vi "SecurityCamera.vi"() -> ()   [LabVIEW 2013]
uses:
  <vilib>/vision/Avi.llb/IMAQ AVI2 Refnum.ctl
  <vilib>/vision/Image Controls.llb/IMAQ Image.ctl
  SecurityCameraStates.ctl
  MouseCarousel-Main/GlobalVariables.vi
panel:
  out "Lost Image Count":u32
  out "Acquired Image":T1
  out "Timestamped Image":T1
  out "Shutdown":bool=TRUE
  out "Exit and Close":bool=TRUE
  in  "stop":bool
  in  "Select Mouse ROI":bool
  in  "Show Mouse ROI":bool
  out "Saving Video":bool=TRUE
  out "FPS":dbl
  out "Close Avi File":bool=TRUE
  out "Open Avi File":bool=TRUE
  out "Lost Frames":u32
  out "Last Image Number":u32
  in  "File Path for Mouse Mask":path=path "C:/PassiveRotationTask/MousePositionMask.bmp"
  out "Mouse mask":T1
  out "Mouse Image":T1(plugin-control)
  out "AVI Refnum - Body":T2
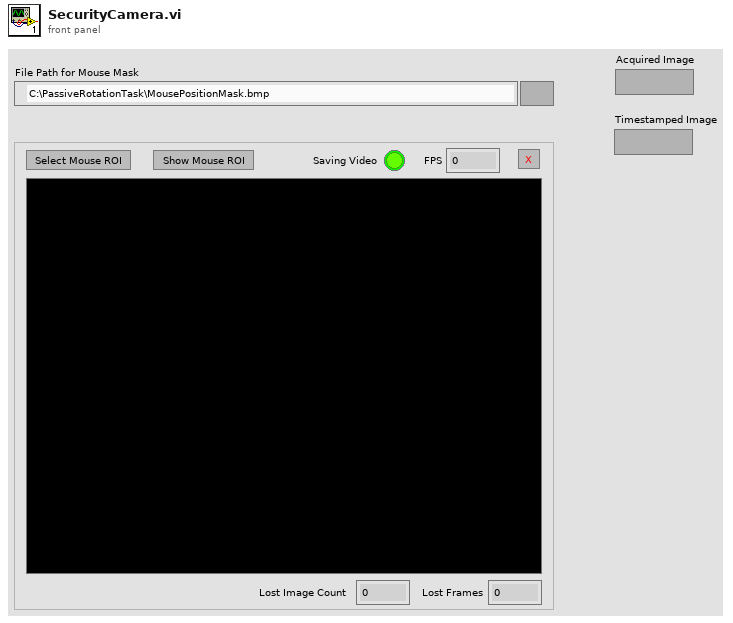
[diagram p1: front panel]
types:
  T1 = typedef "IMAQ Image.ctl" = refnum<image>
  T2 = typedef "IMAQ AVI2 Refnum.ctl" = refnum<k20>
  T3 = typedef "SecurityCameraStates.ctl" = enum16{"Init Security Camera", "Idle", "Process Image", "Acquire Image", "Disconnect Camera", "Exit"}
  T4 = typedef "Image Type" = u32
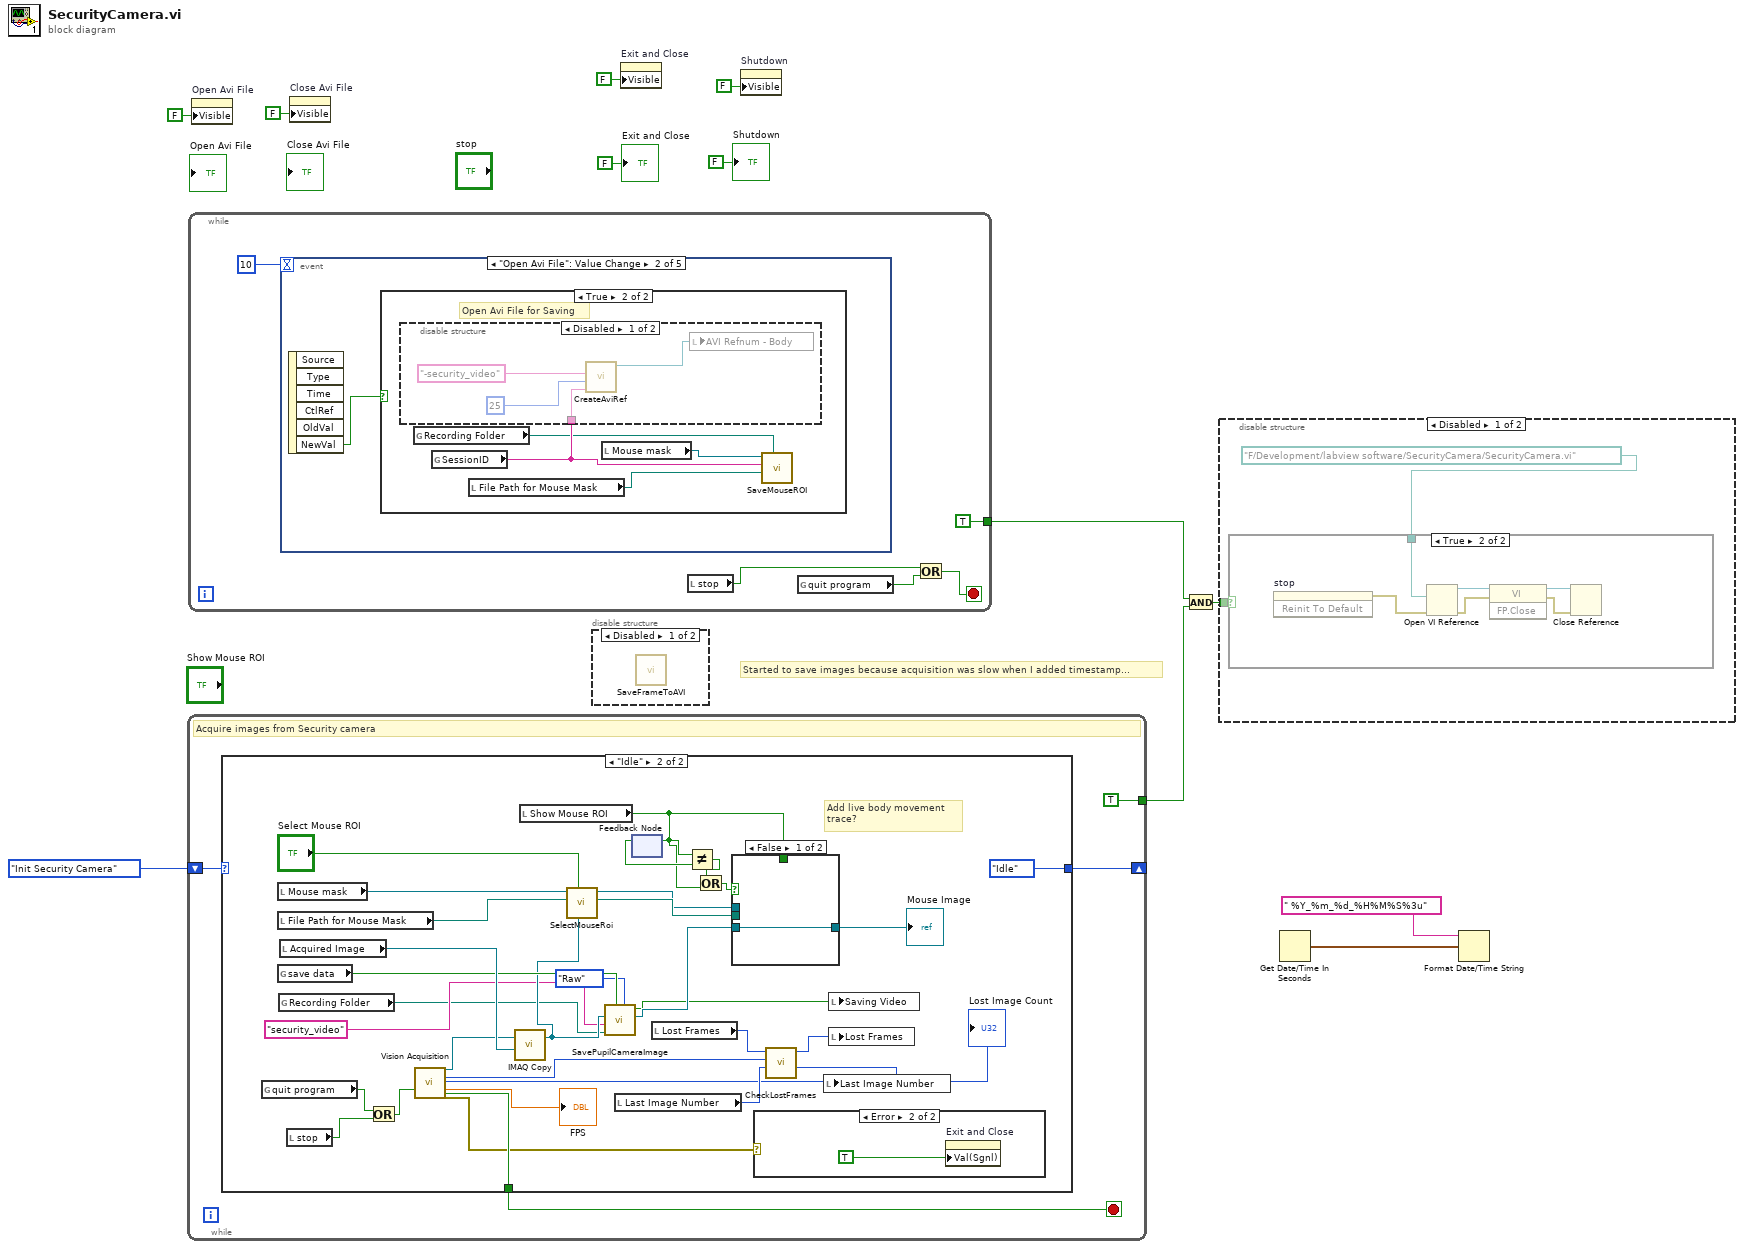
[diagram p0: block diagram]
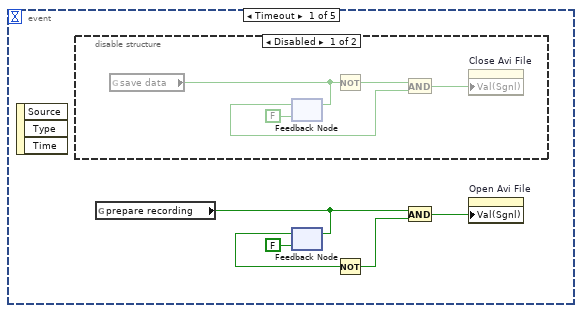
[diagram p5: hidden frame]
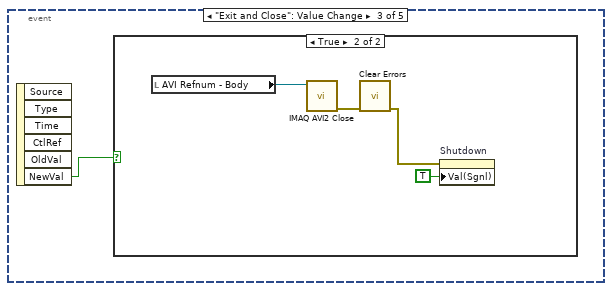
[diagram p9: hidden frame]
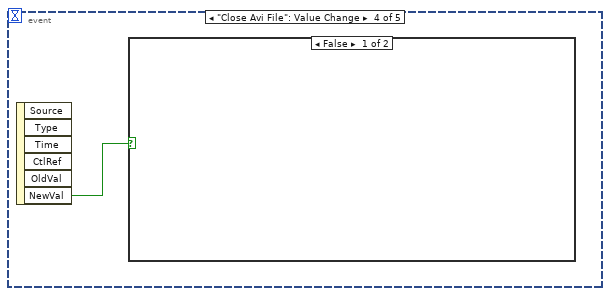
[diagram p11: hidden frame]
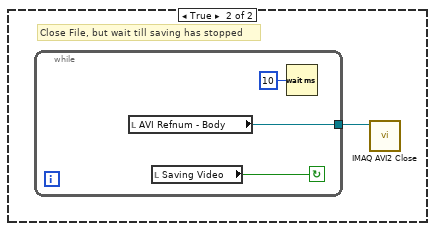
[diagram p12: hidden frame]
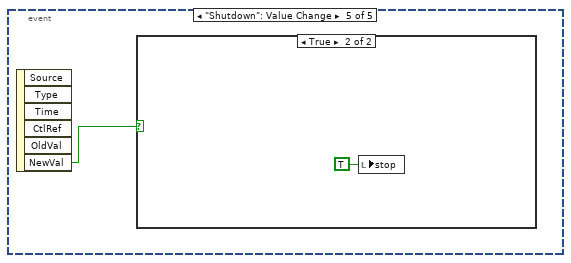
[diagram p13: hidden frame]
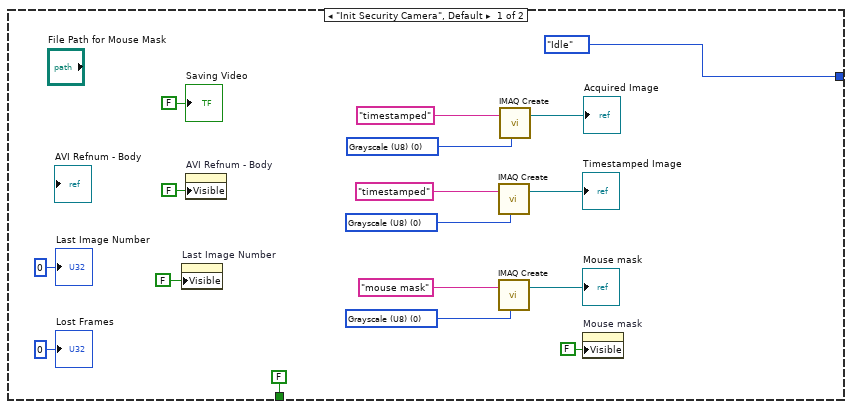
[diagram p15: hidden frame]
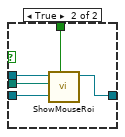
[diagram p16: hidden frame]
diagram:
  # "Started to save images because acquisition was slow when I added timestamp..."
  n1 = while {
    shift-right: [w15] -> _
    shift-left: SecurityCameraStates."Init Security Camera" ("States") -> [w14]
    tunnel: [TRUE] -> w8
    stop <- w16 stop-if-true
    # "Acquire images from Security camera"
    n2 = case shown="\"Idle\"" w14 {
      tunnel: [FALSE ("Stopped") w63] -> w16
      tunnel: [SecurityCameraStates."Idle" ("States") SecurityCameraStates."Idle" ("States")] -> w15
      frame "Init Security Camera", Default {
        w18 = T4 0 items=["Grayscale (U8)", "Grayscale (I16)", "Grayscale (SGL)", "Complex (CSG)", "RGB (U32)", "HSL (U32)", "RGB (U64)", "Grayscale (U16)"] ("Image Type")
        w21 = T4 0 items=["Grayscale (U8)", "Grayscale (I16)", "Grayscale (SGL)", "Complex (CSG)", "RGB (U32)", "HSL (U32)", "RGB (U64)", "Grayscale (U16)"] ("Image Type")
        w25 = T4 0 items=["Grayscale (U8)", "Grayscale (I16)", "Grayscale (SGL)", "Complex (CSG)", "RGB (U32)", "HSL (U32)", "RGB (U64)", "Grayscale (U16)"] ("Image Type")
        n3 = property on="Last Image Number" class="DigNum (strict)"("Visible"=FALSE) -> ()  [unwired: 2 in, 2 out]
        n4 = property on="AVI Refnum - Body" class="IMAQAVI (strict)"("Visible"=FALSE) -> ()  [unwired: 2 in, 2 out]
        n5 = call "IMAQ Create"("Image Name"="timestamped", "Image Type"=w21) -> ("New Image"=→"Timestamped Image":T1)  [unwired: 3 in, 1 out]
        n6 = call "IMAQ Create"("Image Name"="mouse mask", "Image Type"=w25) -> ("New Image"=→"Mouse mask":T1)  [unwired: 3 in, 1 out]
        n7 = call "IMAQ Create"("Image Name"="timestamped", "Image Type"=w18) -> ("New Image"=→"Acquired Image":T1)  [unwired: 3 in, 1 out]
        n8 = property on="Mouse mask" class="IMAQImage (strict)"("Visible"=FALSE) -> ()  [unwired: 2 in, 2 out]
        "Last Image Number" <- u32 0 ("Last Image number 2")
        "Lost Frames" <- u32 0 ("LostFrames 2")
        "Saving Video" <- FALSE ("Saving Security Video")
      }
      frame "Idle" {
        # "Add live body movement\ntrace?"
        n9 = global read "GlobalVariables.vi" "quit program"() -> (w52:bool)
        n10 = local read "Mouse mask"() -> (w59:T1)
        n11 = local read "File Path for Mouse Mask"() -> (w61:path)
        n12 = global read "GlobalVariables.vi" "save data"() -> (w41:bool)
        n13 = global read "GlobalVariables.vi" "Recording Folder"() -> (w37:path)
        n14 = local read "Acquired Image"() -> (w46:T1)
        n15 = local read "stop"() -> (w51:bool)
        n16 = Or(x=w52, y=w51) -> (x .or. y?=w50:bool)
        n17 = call "Vision Acquisition"("Stop (F)"=w50) -> ("Image Out"=w42:T1, "Image Number"=w55:i32, "Lost Image Count"=→"Lost Image Count":u32, "Frame Rate"=→"FPS":dbl, "Stopped"=w63:bool, "error out"=w49:errorcluster)  [unwired: 20 in, 1 out]
        n18 = call "IMAQ Copy"("Image Dst"=w46, "Image Src"=w42) -> ("Image Dst Out"=w39:T1)  [unwired: 4 in, 1 out]
        n19 = local read "Show Mouse ROI"() -> (w43:bool)
        n20 = call "SelectMouseRoi.vi"("Refnum in"=w39, "Select mouse"="Select Mouse ROI", "File Path for Mouse Mask"=w61, "MouseRoi"=w59) -> ()  [unwired: 7 in, 1 out]
        n21 = call "SavePupilCameraImage.vi"("Save Format"=enum16{"Png", "Raw"}."Raw", "Save Image?"=w41, "Block Folder"=w37, "Subfolder"="security_video", "Refnum in"=w39) -> ("Refnum out (duplicate)"=w40:T1, "ImageSaved"=w36:bool)  [unwired: 5 in]
        n22 = local read "Last Image Number"() -> (w54:u32)
        n23 = feedback-in #1(w43) -> ()
        n24 = feedback #1() -> (w47:bool)  [unwired: 1 in]
        n25 = local read "Lost Frames"() -> (w56:u32)
        n26 = Not Equal?(x=w43, y=w47) -> (x != y?=w45:bool)
        n27 = Or(x=w45, y=w43) -> (x .or. y?=w44:bool)
        n28 = case shown="False" w44 {
          tunnel: w61 -> [_ w69]
          tunnel: w40 -> [w64 w68]
          tunnel: w59 -> [_ w67]
          tunnel: [w64 w66] -> w48
          tunnel: w43 -> [_ w65]
          frame False {
          }
          frame True {
            n29 = call "ShowMouseRoi.vi"("Refnum Image In"=w68, "Show mouse selection"=w65, "File Path for Mouse Mask"=w69, "Refnum MouseROI"=w67) -> ("Refnum Image out"=w66:T1)  [unwired: 7 in]
          }
        }
        "Mouse Image" <- w48
        n30 = case shown="Error" w49 {
          frame No Error {
          }
          frame Error {
            n31 = property on="Exit and Close" class="Bool (strict)"("Val(Sgnl)"=TRUE ("Value (Signaling)")) -> ()  [unwired: 2 in, 2 out]
          }
        }
        n32 = call "CheckLostFrames.vi"("Last Image number"=w54, "Image Number"=w55, "LostFrames in"=w56) -> ("Last Image Number"=w57:u32, "LostFrames out"=w58:u32)  [unwired: 5 in, 2 out]
        n33 = local write "Last Image Number"(w57) -> ()
        n34 = local write "Saving Video"(w36) -> ()
        n35 = local write "Lost Frames"(w58) -> ()
      }
    }
  }
  n36 = while {
    tunnel: [TRUE] -> w9
    stop <- w72 stop-if-true
    n37 = event shown="[1] \"Open Avi File\": Value Change" {
      selector: _ -> [_ _ _ _ _]
      dyn-events: _ -> [_ _ _ _ _]
      timeout: 10 -> [_ _ _ _ _]
      event Timeout {
        n38 = event-data() -> ()  [unwired: 1 in, 3 out]
        n39 = disable-structure shown="Disabled" {
          frame Disabled {
            n40 = global read "GlobalVariables.vi" "save data"() -> (w84:bool)
            n41 = feedback #2(FALSE ("save data")) -> (w82:bool)
            n42 = feedback-in #2(w84) -> ()
            n43 = Not(x=w84) -> (.not. x?=w83:bool)
            n44 = And(x=w83, y=w82) -> (x .and. y?=w81:bool)
            n45 = property on="Close Avi File" class="Bool (strict)"("Val(Sgnl)"=w81) -> ()  [unwired: 2 in, 2 out]
          }
          frame Enabled {
          }
        }
        n46 = global read "GlobalVariables.vi" "prepare recording"() -> (w78:bool)
        n47 = feedback #3(FALSE ("save data")) -> (w77:bool)
        n48 = feedback-in #3(w78) -> ()
        n49 = Not(x=w77) -> (.not. x?=w76:bool)
        n50 = And(x=w78, y=w76) -> (x .and. y?=w79:bool)
        n51 = property on="Open Avi File" class="Bool (strict)"("Val(Sgnl)"=w79) -> ()  [unwired: 2 in, 2 out]
      }
      event "Open Avi File": Value Change {
        n52 = event-data() -> ("NewVal"=w86:bool)  [unwired: 1 in, 5 out]
        n53 = case shown="True" w86 {
          frame False {
          }
          frame True {
            # "Open Avi File for Saving"
            n54 = global read "GlobalVariables.vi" "Recording Folder"() -> (w87:path)
            n55 = global read "GlobalVariables.vi" "SessionID"() -> (w88:string)
            n56 = disable-structure shown="Disabled" {
              disable-tunnel: w88 -> [w91 _]
              frame Disabled {
                n57 = call "CreateAviRef.vi"("sessionID"=w91, "Framerate"=u32 25, "Filename prefix"="-security_video") -> ("Refnum out"=w93:T2, "Block folder"=w92:path)  [unwired: 7 in]
                n58 = local write "AVI Refnum - Body"(w93) -> ()
              }
              frame Enabled {
              }
            }
            n59 = local read "File Path for Mouse Mask"() -> (w90:path)
            n60 = local read "Mouse mask"() -> (w89:T1)
            n61 = call "SaveMouseROI.vi"("BlockFolderPath"=w87, "File Path for Mouse Mask"=w90, "sessionID"=w88, "MouseRoi Refnum in"=w89) -> ()  [unwired: 8 in]
          }
        }
      }
      event "Exit and Close": Value Change {
        n62 = event-data() -> ("NewVal"=w96:bool)  [unwired: 1 in, 5 out]
        n63 = case shown="True" w96 {
          frame False {
          }
          frame True {
            n64 = local read "AVI Refnum - Body"() -> (w100:T2)
            n65 = call "IMAQ AVI2 Close"("AVI Refnum"=w100) -> ("error out"=w99:errorcluster)  [unwired: 10 in]
            n66 = call <vilib>:"Clear Errors.vi"("error in (no error)"=w99) -> ("error out"=w98:errorcluster)  [unwired: 6 in]
            n67 = property on="Shutdown" class="Bool (strict)"(error in=w98, "Val(Sgnl)"=TRUE ("Value (Signaling)")) -> ()  [unwired: 1 in, 2 out]
          }
        }
      }
      event "Close Avi File": Value Change {
        n68 = event-data() -> ("NewVal"=w101:bool)  [unwired: 1 in, 5 out]
        n69 = case shown="False" w101 {
          frame False {
          }
          frame True {
            # "Close File, but wait till saving has stopped"
            n70 = while {
              tunnel: [w103] -> w102
              stop <- w105 continue-if-true
              n71 = local read "AVI Refnum - Body"() -> (w103:T2)
              n72 = local read "Saving Video"() -> (w105:bool)
              n73 = Wait (ms)(milliseconds to wait=u32 10) -> ()  [unwired: 1 out]
            }
            n74 = call "IMAQ AVI2 Close"("AVI Refnum"=w102) -> ()  [unwired: 10 in, 1 out]
          }
        }
      }
      event "Shutdown": Value Change {
        n75 = event-data() -> ("NewVal"=w106:bool)  [unwired: 1 in, 5 out]
        n76 = case shown="True" w106 {
          frame False {
          }
          frame True {
            n77 = local write "stop"(TRUE ("stop")) -> ()
          }
        }
      }
    }
    n78 = local read "stop"() -> (w73:bool)
    n79 = global read "GlobalVariables.vi" "quit program"() -> (w74:bool)
    n80 = Or(x=w73, y=w74) -> (x .or. y?=w72:bool)
  }
  n81 = property on="Open Avi File" class="Bool (strict)"("Visible"=FALSE) -> ()  [unwired: 2 in, 2 out]
  n82 = property on="Close Avi File" class="Bool (strict)"("Visible"=FALSE) -> ()  [unwired: 2 in, 2 out]
  n83 = disable-structure shown="Disabled" {
    frame Disabled {
      n84 = call "SaveFrameToAVI.vi"() -> ()  [unwired: 10 in, 2 out]
    }
    frame Enabled {
    }
  }
  n85 = property on="Exit and Close" class="Bool (strict)"("Visible"=FALSE) -> ()  [unwired: 2 in, 2 out]
  n86 = property on="Shutdown" class="Bool (strict)"("Visible"=FALSE) -> ()  [unwired: 2 in, 2 out]
  n87 = And(x=w9, y=w8) -> (x .and. y?=w7:bool)
  n88 = disable-structure shown="Disabled" {
    disable-tunnel: w7 -> [w109 _]
    frame Disabled {
      n89 = case shown="True" w109 {
        tunnel: path "F:/Development/labview software/SecurityCamera/SecurityCamera.vi" ("vi path") -> [_ w110]
        frame False {
        }
        frame True {
          n90 = invoke on="stop" class="Bool (strict)" method="Reinit To Default"() -> (error out=w113:errorcluster)  [unwired: 3 in, 2 out]
          n91 = Open VI Reference(vi path=w110, error in (no error)=w113) -> (vi reference=w115:refnum<vi>, error out=w112:errorcluster)  [unwired: 4 in]
          n92 = invoke class="VI" method="FP.Close"(reference=w115, error in=w112) -> (reference out=w114:refnum<vi>, error out=w111:errorcluster)  [unwired: 1 in, 1 out]
          n93 = Close Reference(reference=w114, error in (no error)=w111) -> ()  [unwired: 1 out]
        }
      }
    }
    frame Enabled {
    }
  }
  n94 = Get Date/Time In Seconds() -> (seconds since 1Jan1904=w1:timestamp)
  n95 = Format Date/Time String(time format string (%c)=" %Y_%m_%d_%H%M%S%3u", seconds (now)=w1) -> ()  [unwired: 1 in, 1 out]
  "Exit and Close" <- FALSE ("Exit and Close")
  "Shutdown" <- FALSE ("Shutdown")
